vi "solar_qtimer Set Stop All.vi"(6 "Suppress Errors? (T)":bool=TRUE, 8 "error in (no error)":errorcluster, 11 "QTimer Refnum in":T1) -> (0 "error out":errorcluster, 1 "Previously Running":bool[](array[boolean]), 2 "QTimers":string[](array[string]), 3 "QTimer Refnum out":T1)   [LabVIEW 2018]
doc: "This stops all registered QTimers from executing."
uses:
  solar_qtimer_ctl Refnum.ctl
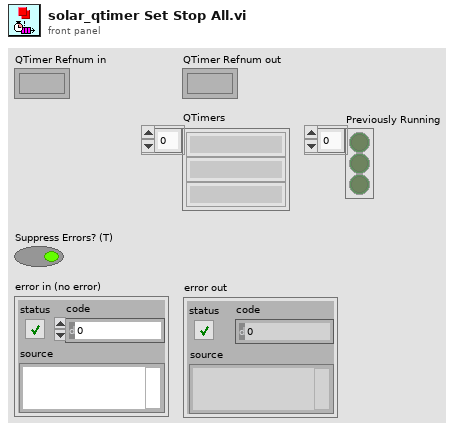
[diagram p1: front panel]
types:
  T1 = typedef "solar_qtimer_ctl Refnum.ctl" = refnum<k1>
  T2 = typedef "solar_qtimer_ctl SEQ.ctl" = cluster{"QTimers":T3[]}
  T3 = typedef "solar_qtimer_ctl QTimer.ctl" = cluster{"Settings":T4, "Queue":refnum<queue>, "QTimerQ":refnum<queue>, "VI Refnum":refnum<vi>}
  T4 = typedef "solar_qtimer_ctl QTimer Settings.ctl" = cluster{"QTimer":string, "Delay":i32, "Start":bool, "EnQ_Type":enum8{"Normal", "Priority", "IgnoreIfExists"}, "Messages":cluster{"MSG":string, "DATA":variant}[]}
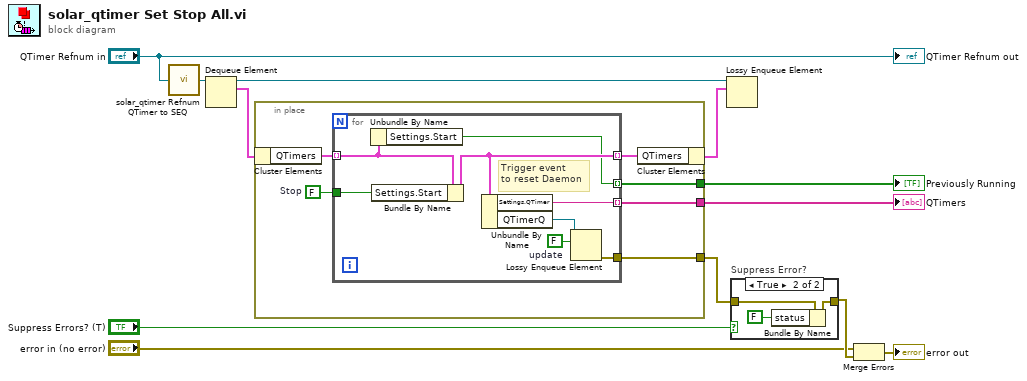
[diagram p0: block diagram]
diagram:
  n1 = call "solar_qtimer Refnum QTimer to SEQ.vi"("QTimer Refnum"="QTimer Refnum in") -> ("QTimers SEQ"=w11:refnum<queue>)
  n2 = Dequeue Element(queue=w11) -> (queue out=w10:refnum<queue>, element=w9:T2)  [unwired: 2 in, 2 out]
  n3 = in-place {
    in-place-border: [w16] -> w5
    in-place-border: [w14] -> w2
    in-place-border: [w13] -> w1
    w15 = FALSE  # Stop
    n4 = in-place-cluster #1(w9) -> ("QTimers"=w18:T3[])
    n5 = for {
      tunnel: [w21] -> w16
      tunnel: w15 -> [w26]
      tunnel: w18 -> [w23] mode=indexing
      tunnel: [w24] -> w17 mode=indexing
      tunnel: [w25] -> w14 mode=indexing
      tunnel: [w22] -> w13 mode=indexing
      w19 = FALSE  # update
      # "Trigger event\nto reset Daemon"
      n6 = Unbundle By Name(w23) -> ("Settings.Start"=w22:bool)
      n7 = Bundle By Name(cluster=w23, "Settings.Start"=w26) -> (w24:T3)
      n8 = Unbundle By Name(w24) -> ("Settings.QTimer"=w25:string, "QTimerQ"=w20:refnum<queue>)
      n9 = Lossy Enqueue Element(queue=w20, element=w19) -> (error out=w21:errorcluster)  [unwired: 1 in, 3 out]
    }
    n10 = in-place-cluster #1("QTimers"=w17) -> (w8:T2)
  }
  "QTimers" <- w2
  "Previously Running" <- w1
  n11 = Lossy Enqueue Element(queue=w10, element=w8) -> ()  [unwired: 1 in, 4 out]
  n12 = case "Suppress Error?" shown="True" "Suppress Errors? (T)" {
    tunnel: w5 -> [w27 w30]
    tunnel: [w27 w29] -> w6
    frame False {
    }
    frame True {
      n13 = Bundle By Name(cluster=w30, "status"=FALSE) -> (w29:errorcluster)
    }
  }
  n14 = Merge Errors("error in (no error)", w6) -> (→"error out":errorcluster)
  "QTimer Refnum out" <- "QTimer Refnum in"
